vi "Error Query.vi"(8 "error in (no error)":errorcluster, 10 "Command Type (0)":i32, 11 "VISA resource name":refnum<visa-resource-name>) -> (0 "error out":errorcluster, 1 "Error Message":string, 2 "Error Code":i16, 3 "VISA resource name out":refnum<visa-resource-name>)   [LabVIEW 2018, in "LTB-1.lvlib" / "3150.lvlib"]
doc: "This VI queries the error/event queue for the next item and removes it from the queue. \n\nQueries the instrument for any errors in the instrument's error queue. It will continue to read errors until all errors have been read from the instrument. The response message consists of two fields separated into <Error Code> and <Error Message>. \nError out will contain the error/warnings generated during the execution with RS-232 or GPIB mode of communication and will be visible through the low-level driver VI's/Examples.\n\n<B>Note:</B>\nThis VI is called automatically by most driver VIs so it is not usually necessary to call this in an application."
uses:
  3150.lvlib
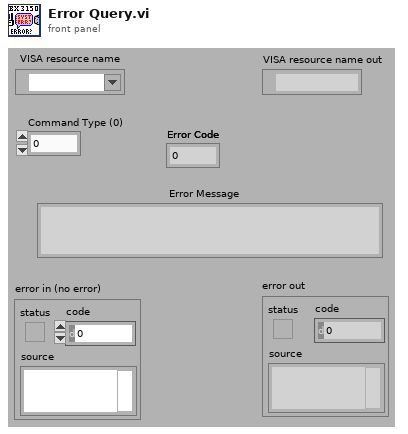
[diagram p1: front panel]
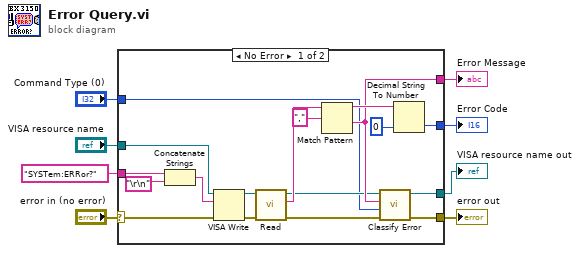
[diagram p0: block diagram]
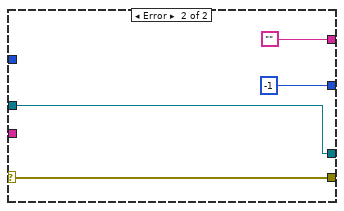
[diagram p2: hidden frame]
diagram:
  n1 = case shown="No Error" "error in (no error)" {
    selector: "error in (no error)" -> [w19 w29]
    tunnel: "VISA resource name" -> [w23 w27]
    tunnel: "SYSTem:ERRor?" ("Command") -> [w10 _]
    tunnel: [w12 w29] -> w6
    tunnel: [w24 -1] -> w4
    tunnel: [w17 ""] -> w3
    tunnel: [w15 w27] -> w2
    tunnel: "Command Type (0)" -> [w14 _]
    frame No Error {
      n2 = Concatenate Strings(w10, "\r\n") -> (w9:string)
      n3 = VISA Write(VISA resource name=w23, write buffer=w9, error in (no error)=w19) -> (VISA resource name out=w22:refnum<visa-resource-name>, error out=w21:errorcluster)  [unwired: 1 out]
      n4 = call "Read.vi"("error in (no error)"=w21, "VISA resource name"=w22) -> ("error out"=w13:errorcluster, "Message Received"=w20:string, "VISA resource name out"=w16:refnum<visa-resource-name>)  [unwired: 7 out]
      n5 = Match Pattern(string=w20, regular expression="," ("search string/char (-)")) -> (before substring=w25:string, after substring=w17:string)  [unwired: 3 out]
      n6 = call "Classify Error.vi"("error in (no error)"=w13, "Command Type (0)"=w14, "Message String"=w17, "VISA resource name"=w16) -> ("error out"=w12:errorcluster, "VISA resource name out"=w15:refnum<visa-resource-name>)  [unwired: 6 out]
      n7 = Decimal String To Number(string=w25, default (0L)=0 ("default (0 I32)")) -> (number=w24:i32)  [unwired: 2 out]
    }
    frame Error {
    }
  }
  "VISA resource name out" <- w2
  "error out" <- w6
  "Error Code" <- w4
  "Error Message" <- w3
